vi "manualPD.vi"(10 "Use DDS display equivalent?":bool, 11 "Manual Photodiode (V)":dbl) -> (2 "DDS display value":u16, 3 "Photodiode string out":string)   [LabVIEW 2012, in "DDS9954_v2013.lvlib"]
uses:
  DDS9954_v2013.lvlib
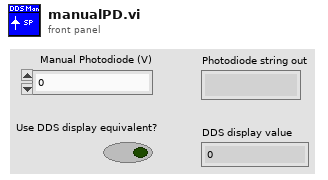
[diagram p1: front panel]
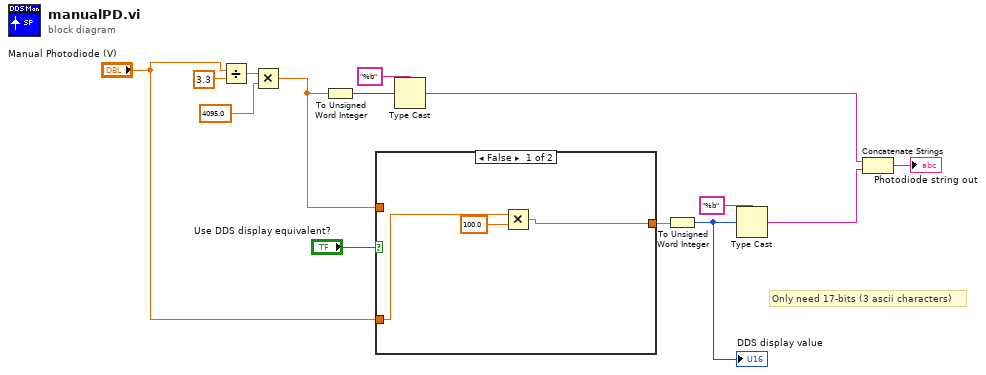
[diagram p0: block diagram]
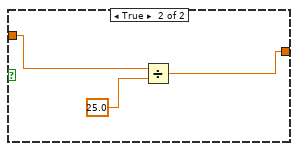
[diagram p2: hidden frame]
diagram:
  # "Only need 17-bits (3 ascii characters)"
  n1 = Divide(x="Manual Photodiode (V)", y=3.3) -> (x/y=w4:dbl)
  n2 = Multiply(x=w4, y=4095.0) -> (x*y=w1:dbl)
  n3 = To Unsigned Word Integer(number=w1) -> (unsigned 16bit integer=w14:u16)
  n4 = case shown="False" "Use DDS display equivalent?" {
    tunnel: w1 -> [_ w20]
    tunnel: "Manual Photodiode (V)" -> [w17 _]
    tunnel: [w15 w18] -> w9
    frame False {
      n5 = Multiply(x=w17, y=100.0) -> (x*y=w15:dbl)
    }
    frame True {
      n6 = Divide(x=w20, y=25.0) -> (x/y=w18:dbl)
    }
  }
  n7 = Type Cast(type="%b", x=w14) -> (*(type *) &x=w8:string)
  n8 = To Unsigned Word Integer(number=w9) -> (unsigned 16bit integer=w11:u16)
  "DDS display value" <- w11
  n9 = Type Cast(type="%b", x=w11) -> (*(type *) &x=w6:string)
  n10 = Concatenate Strings(w8, w6) -> (→"Photodiode string out":string)
